vi "CRYStep Update.vi"(5 "sOption":string, 6 "SequenceTree":refnum<vi>, 7 "StepName":string, 8 "Step Name Write":bool, 9 "Seq-step setup":string, 10 "Proper VI No":i32, 11 "StepIdentifier":string) -> ()   [LabVIEW 2013]
uses:
  CRYSystem/Calibration/SubVI/CRYCal Global.vi
  CRYProject Editor Global.vi
panel:
  in  "Name/Identifier":bool
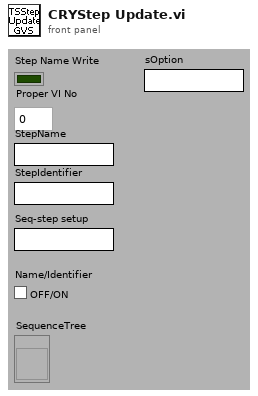
[diagram p1: front panel]
types:
  T1 = typedef "CRYTS.ctl" = cluster{"No.TS":u16, "TS File Path":path, "TS Name":string, "EditStepName":string, "Steps":T2[], "New State":bool, "Change State":bool, "Flattened CurveLib Data":string, "Document Data":string, "EditStepNo":u16, "Operator Start File":string, "Sequence Type":string, "Sequence Language":string}
  T2 = typedef "CRYStep.ctl" = cluster{"No.VI":i32, "Category":string, "StepName":string, "Seq setup flattened":string, "Comment":string, "Steps config.":bool[], "Jump config":i32[], "Start":dbl, "Increment":dbl, "Name":string, "Unit":string, "Y data":u16, "Y prefix":string, "Y dB ref":dbl, "Y unit":string, "Repeat State Array":cluster{"Start":dbl, "Increment":dbl, "Count":i32, "Num":i32}[]}
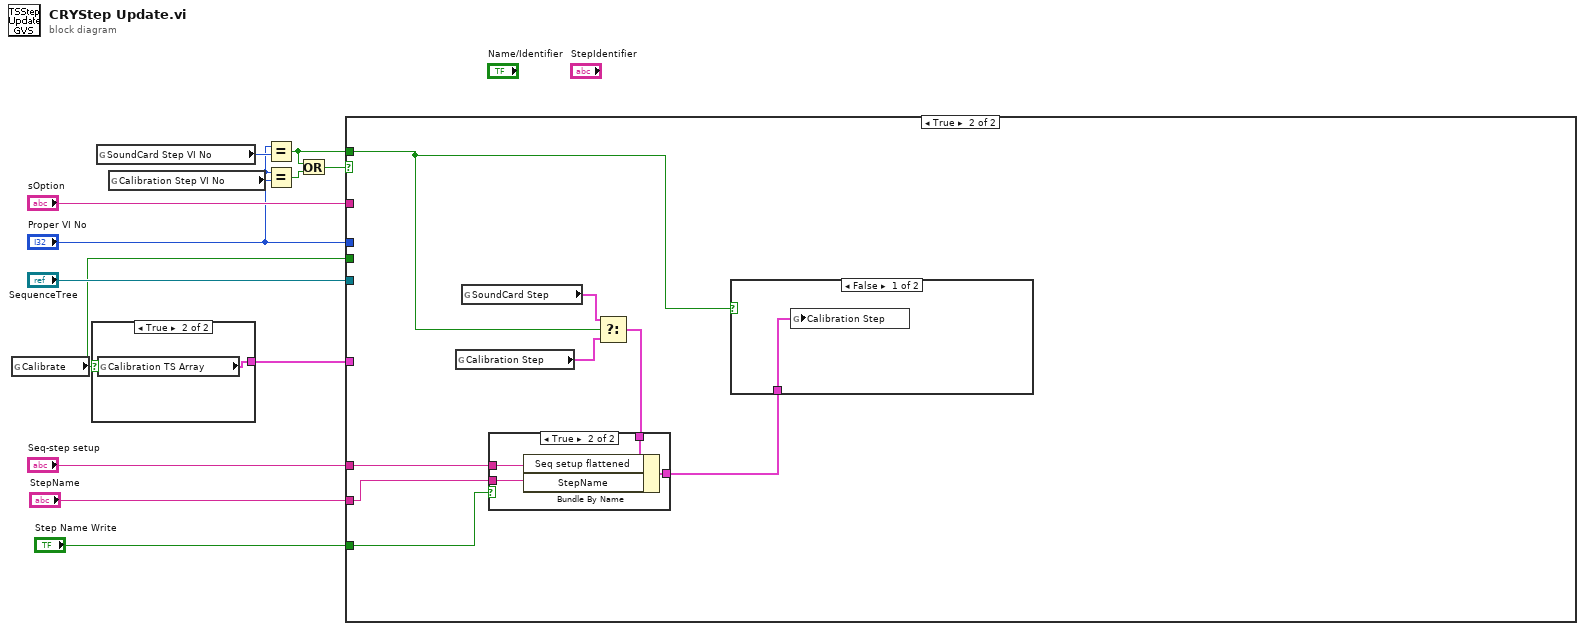
[diagram p0: block diagram]
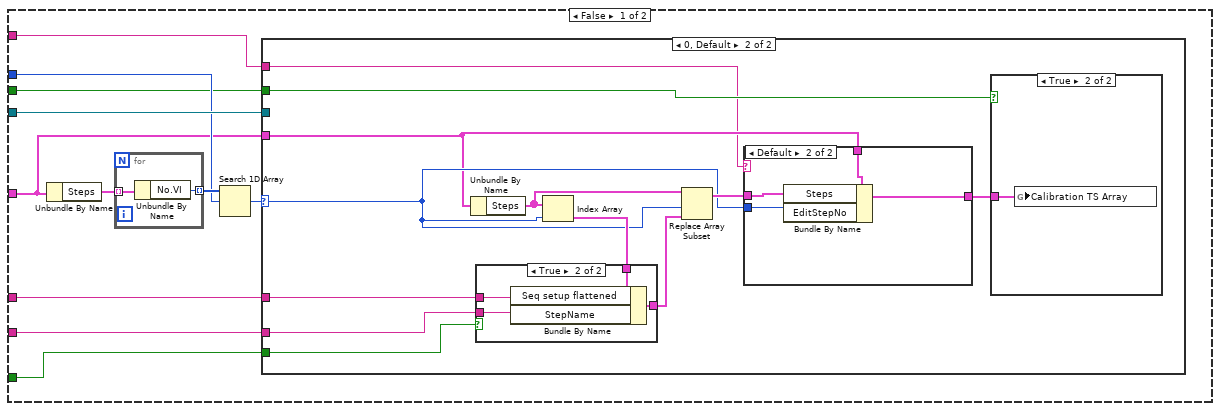
[diagram p2: hidden frame]
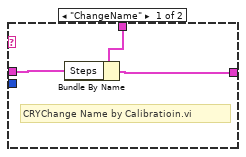
[diagram p4: hidden frame]
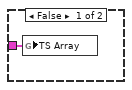
[diagram p5: hidden frame]
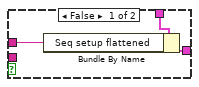
[diagram p6: hidden frame]
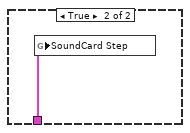
[diagram p7: hidden frame]
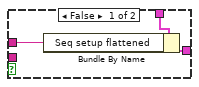
[diagram p8: hidden frame]
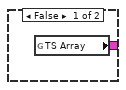
[diagram p9: hidden frame]
diagram:
  n1 = global read "CRYCal Global.vi" "Calibrate"() -> (w8:bool)
  n2 = case shown="True" w8 {
    tunnel: [w14 w15] -> w9
    frame False {
      n3 = global read "CRYProject Editor Global.vi" "TS Array"() -> (w14:T1)
    }
    frame True {
      n4 = global read "CRYProject Editor Global.vi" "Calibration TS Array"() -> (w15:T1)
    }
  }
  n5 = global read "CRYProject Editor Global.vi" "SoundCard Step VI No"() -> (w6:i32)
  n6 = global read "CRYProject Editor Global.vi" "Calibration Step VI No"() -> (w5:i32)
  n7 = Equal?(x="Proper VI No", y=w6) -> (x = y?=w1:bool)
  n8 = Equal?(x="Proper VI No", y=w5) -> (x = y?=w3:bool)
  n9 = Or(x=w1, y=w3) -> (x .or. y?=w2:bool)
  n10 = case shown="True" w2 {
    tunnel: "SequenceTree" -> [w26 _]
    tunnel: "Seq-step setup" -> [w25 w64]
    tunnel: "Proper VI No" -> [w21 _]
    tunnel: "StepName" -> [w20 w63]
    tunnel: "Step Name Write" -> [w19 w62]
    tunnel: w9 -> [w18 _]
    tunnel: w8 -> [w17 _]
    tunnel: "sOption" -> [w16 _]
    tunnel: w1 -> [_ w57]
    frame False {
      n11 = Unbundle By Name(w18) -> ("Steps"=w23:T2[])
      n12 = for {
        tunnel: w23 -> [w56] mode=indexing
        tunnel: [w55] -> w22 mode=indexing
        n13 = Unbundle By Name(w56) -> ("No.VI"=w55:i32)
      }
      n14 = Search 1D Array(1D array=w22, element=w21) -> (index of element=w24:i32)  [unwired: 1 out]
      n15 = case shown="0, Default" w24 {
        selector: w24 -> [_ w30]
        tunnel: w26 -> [_ _]
        tunnel: w25 -> [_ w37]
        tunnel: w20 -> [_ w32]
        tunnel: w19 -> [_ w31]
        tunnel: w18 -> [_ w29]
        tunnel: w17 -> [_ w28]
        tunnel: w16 -> [_ w27]
        frame -1 {
        }
        frame 0, Default {
          n16 = Unbundle By Name(w29) -> ("Steps"=w36:T2[])
          n17 = Index Array(array=w36, index=w30) -> (element=w38:T2)
          n18 = case shown="True" w31 {
            tunnel: w38 -> [w50 w54]
            tunnel: w37 -> [w49 w53]
            tunnel: [w48 w52] -> w35
            tunnel: w32 -> [_ w51]
            frame False {
              n19 = Bundle By Name(cluster=w50, "Seq setup flattened"=w49) -> (w48:T2)
            }
            frame True {
              n20 = Bundle By Name(cluster=w54, "Seq setup flattened"=w53, "StepName"=w51) -> (w52:T2)
            }
          }
          n21 = Replace Array Subset(array=w36, new element=w35, index=w30) -> (w34:T2[])
          n22 = case shown="Default" w27 {
            tunnel: w34 -> [w41 w45]
            tunnel: [w40 w44] -> w33
            tunnel: w30 -> [_ w43]
            tunnel: w29 -> [w39 w42]
            frame "ChangeName" {
              # "CRYChange Name by Calibratioin.vi"
              n23 = Bundle By Name(cluster=w39, "Steps"=w41) -> (w40:T1)
            }
            frame Default {
              n24 = Bundle By Name(cluster=w42, "Steps"=w45, "EditStepNo"=w43) -> (w44:T1)
            }
          }
          n25 = case shown="True" w28 {
            tunnel: w33 -> [w46 w47]
            frame False {
              n26 = global write "CRYProject Editor Global.vi" "TS Array"(w46) -> ()
            }
            frame True {
              n27 = global write "CRYProject Editor Global.vi" "Calibration TS Array"(w47) -> ()
            }
          }
        }
      }
    }
    frame True {
      n28 = global read "CRYProject Editor Global.vi" "Calibration Step"() -> (w60:T2)
      n29 = global read "CRYProject Editor Global.vi" "SoundCard Step"() -> (w61:T2)
      n30 = Select(t=w61, s=w57, f=w60) -> (s? t:f=w59:T2)
      n31 = case shown="True" w62 {
        tunnel: w59 -> [w69 w73]
        tunnel: w64 -> [w68 w72]
        tunnel: [w67 w71] -> w58
        tunnel: w63 -> [_ w70]
        frame False {
          n32 = Bundle By Name(cluster=w69, "Seq setup flattened"=w68) -> (w67:T2)
        }
        frame True {
          n33 = Bundle By Name(cluster=w73, "Seq setup flattened"=w72, "StepName"=w70) -> (w71:T2)
        }
      }
      n34 = case shown="False" w57 {
        tunnel: w58 -> [w65 w66]
        frame False {
          n35 = global write "CRYProject Editor Global.vi" "Calibration Step"(w65) -> ()
        }
        frame True {
          n36 = global write "CRYProject Editor Global.vi" "SoundCard Step"(w66) -> ()
        }
      }
    }
  }
